vi "Check Value.vi"(6 "Coerce Value? (F)":bool, 7 "Column Configuration":refnum<class "Column Configuration.lvclass">, 8 "error in (no error)":errorcluster, 9 "Value Type":refnum<class "Value Type.lvclass">, 10 "Value":variant, 11 "Autoincrement in":refnum<class "Autoincrement.lvclass">) -> (0 "error out":errorcluster, 2 "Value Out":variant, 3 "Autoincrement out":refnum<class "Autoincrement.lvclass">)   [LabVIEW 2020, in "Composed Columns.lvlib" / "Autoincrement.lvclass"]
uses:
  Autoincrement.lvclass
  Value Type/Value Type.lvclass
  Basic Columns/Column Configuration/Basic Column Configuration Class/Column Configuration.lvclass
  Numeric Value/Numeric Value.lvclass
  C:/Users/User/Desktop/Raman Program/Database OOP/source/Database OOP/Column Libraries/Value Type/Value Type.lvclass
  Database Libraries/Database Interfaces/Database Interface Class/Database Interface.lvclass
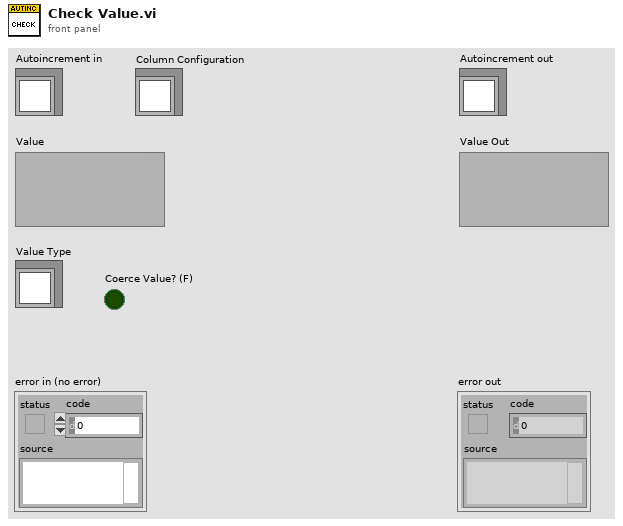
[diagram p1: front panel]
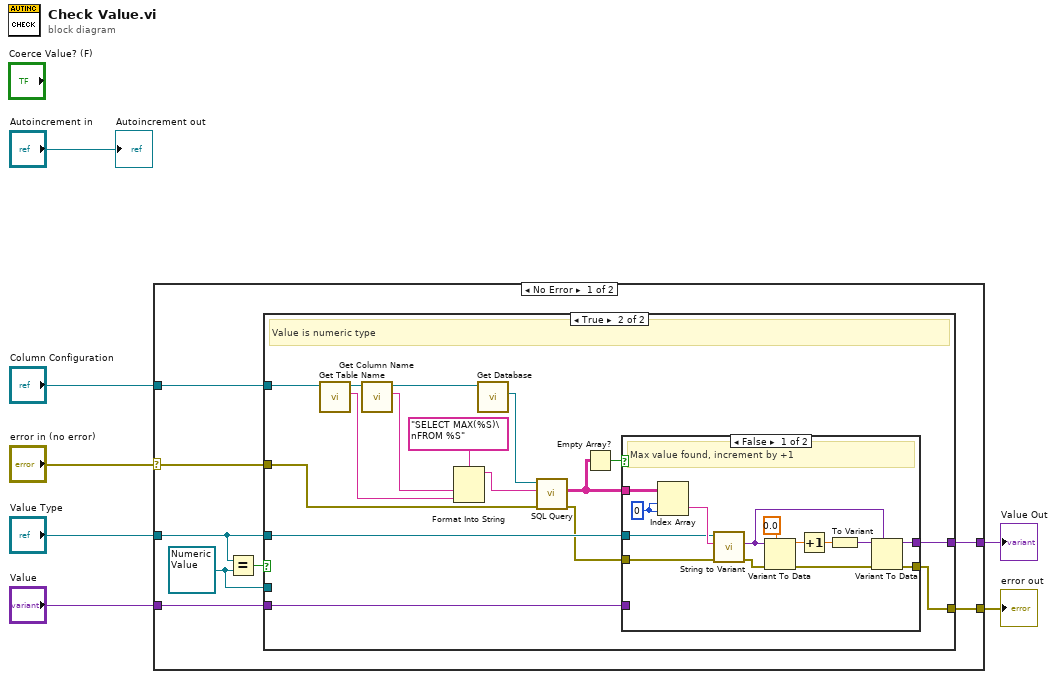
[diagram p0: block diagram]
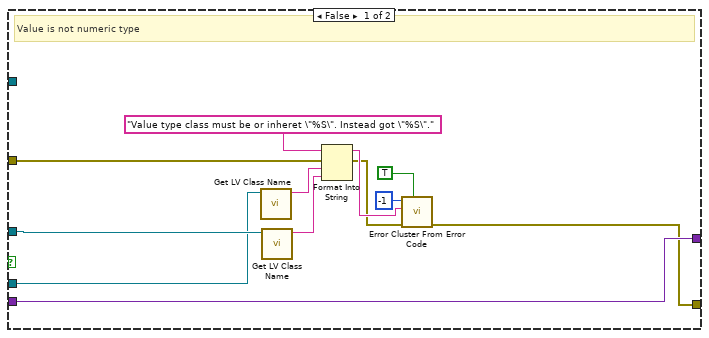
[diagram p2: hidden frame]
diagram:
  n1 = case shown="No Error" "error in (no error)" {
    selector: "error in (no error)" -> [w12 w61]
    tunnel: [w10 w61] -> w5
    tunnel: "Value Type" -> [w9 _]
    tunnel: "Value" -> [w13 w60]
    tunnel: "Column Configuration" -> [w14 _]
    tunnel: [w11 w60] -> w1
    frame No Error {
      w8 = refnum<class "Numeric Value.lvclass"> refnum ("Composed Columns.lvlib:Numeric Value.lvclass")
      n2 = Equal?(x=w9, y=w8) -> (x = y?=w15:bool)
      n3 = case shown="True" w15 {
        tunnel: w14 -> [_ w42]
        tunnel: w9 -> [w25 w33]
        tunnel: w13 -> [w27 w32]
        tunnel: w12 -> [w18 w31]
        tunnel: [w27 w29] -> w11
        tunnel: [w16 w28] -> w10
        tunnel: w8 -> [w24 _]
        frame False {
          # "Value is not numeric type"
          n4 = call <vilib>:"Get LV Class Name.vi"("object"=w24) -> ("class name"=w23:string)  [unwired: 9 in, 1 out]
          n5 = call <vilib>:"Get LV Class Name.vi"("object"=w25) -> ("class name"=w22:string)  [unwired: 9 in, 1 out]
          n6 = Format Into String(format string="Value type class must be or inheret \"%S\". Instead got \"%S\".", error in=w18, w23, w22) -> (resulting string=w19:string, error out=w17:errorcluster)  [unwired: 1 in]
          n7 = call <vilib>:"Error Cluster From Error Code.vi"("show call chain? (False)"=TRUE, "error in (no error)"=w17, "error message (\"\")"=w19, "error code (0)"=-1) -> ("error out"=w16:errorcluster)  [unwired: 5 in]
        }
        frame True {
          # "Value is numeric type"
          n8 = call-dynamic "Get Table Name.vi"("Basic Column Configuration in"=w42) -> ("Table Name"=w41:string, "Basic Column Configuration out"=w39:refnum<class "Column Configuration.lvclass">)  [unwired: 8 in, 1 out]
          n9 = call-dynamic "Get Column Name.vi"("Basic Column Configuration in"=w39) -> ("Column Name"=w40:string, "Basic Column Configuration out"=w38:refnum<class "Column Configuration.lvclass">)  [unwired: 8 in, 1 out]
          n10 = Format Into String(format string="SELECT MAX(%S)\nFROM %S", w40, w41) -> (resulting string=w36:string)  [unwired: 2 in, 1 out]
          n11 = call-dynamic "Get Database.vi"("Basic Column Configuration in"=w38) -> ("Database"=w37:refnum<class "Database Interface.lvclass">)  [unwired: 8 in, 2 out]
          n12 = call-dynamic "SQL Query.vi"("error in (no error)"=w31, "SQL Query"=w36, "Database Interface in"=w37) -> ("error out"=w30:errorcluster, "Query Result"=w35:string[][])  [unwired: 6 in, 1 out]
          n13 = Empty Array?(array=w35) -> (empty?=w34:bool)
          n14 = case shown="False" w34 {
            tunnel: w35 -> [w56 _]
            tunnel: w33 -> [w54 _]
            tunnel: w32 -> [_ w59]
            tunnel: w30 -> [w53 w58]
            tunnel: [w45 w59] -> w29
            tunnel: [w44 w58] -> w28
            frame False {
              w57 = 0 ("index (row)")
              # "Max value found, increment by +1"
              n15 = Index Array(array=w56, index (row)=w57, index (col)=w57) -> (element=w55:string)
              n16 = call-dynamic "String to Variant.vi"("error in (no error)"=w53, "String"=w55, "Value Type in"=w54) -> ("error out"=w52:errorcluster, "Variant"=w47:variant)  [unwired: 6 in, 1 out]
              n17 = Variant To Data(error in=w52, type=0.0, Variant=w47) -> (data=w50:dbl, error out=w46:errorcluster)
              n18 = Increment(x=w50) -> (x+1=w49:dbl)
              n19 = To Variant(anything=w49) -> (Variant=w48:variant)
              n20 = Variant To Data(error in=w46, type=w47, Variant=w48) -> (data=w45:variant, error out=w44:errorcluster)
            }
            frame True {
              # "No max value (error or empty table)"
            }
          }
        }
      }
    }
    frame Error {
    }
  }
  "error out" <- w5
  "Value Out" <- w1
  "Autoincrement out" <- "Autoincrement in"
